vi "Builds Directory.vi"() -> (0 "Builds Directory":path)   [LabVIEW 2017, in "Scripts.lvlib"]
doc: "Gets the \"builds\" directory relative to the project root."
uses:
  Scripts.lvlib
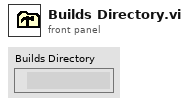
[diagram p1: front panel]
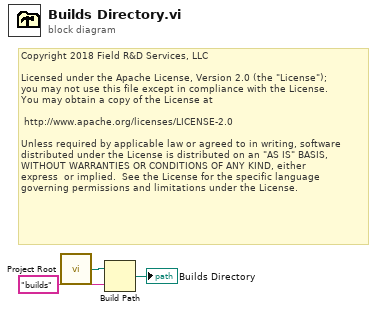
[diagram p0: block diagram]
diagram:
  # "Copyright 2018 Field R&D Services, LLC\n\nLicensed under the Apache License, Version 2.0 (the \"License\");\nyou may not use this file except in compliance with the License.\nYou may obtain a copy of the License at\n\n\thttp://www.apache.org/licenses/LICENSE-2.0\n\nUnless required by applicable law or agreed to in writing, software\ndistributed under the License is distributed on an \"AS IS\" BASIS,\nWITHOUT WARRANTIES OR CONDITIONS OF ANY KIND, either \nexpress  or implied.  See the License for the specific language \ngoverning permissions and limitations under the License."
  n1 = call "Project Root.vi"() -> ("Project Root"=w1:path)
  n2 = Build Path(base path=w1, name or relative path="builds") -> (appended path=→"Builds Directory":path)
